vi "Write Result.vi"(0 "Vector Path in":refnum<class "Vector Abstract Path.lvclass">, 11 "error in (no error)":errorcluster) -> (4 "Vector Path out":refnum<class "Vector Abstract Path.lvclass">, 15 "error out":errorcluster)   [LabVIEW 2023, in "RFFixtureCharact.Public.lvlib" / "Vector Abstract Path.lvclass"]
uses:
  Vector Abstract Path.lvclass
  Common/Result Accessor/Result Accessor.lvclass
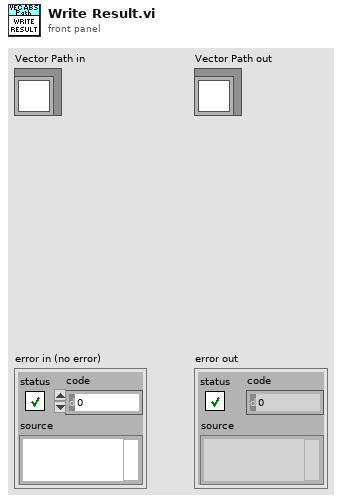
[diagram p1: front panel]
types:
  T1 = typedef "RFFixtureCharact.Public.lvlib/Vector Abstract Path.lvclass/Vector Charact Result.ctl" = cluster{"Port Power":dbl, "Frequency":dbl, "S Parameters":cdb[], "Out Of Limit":bool}
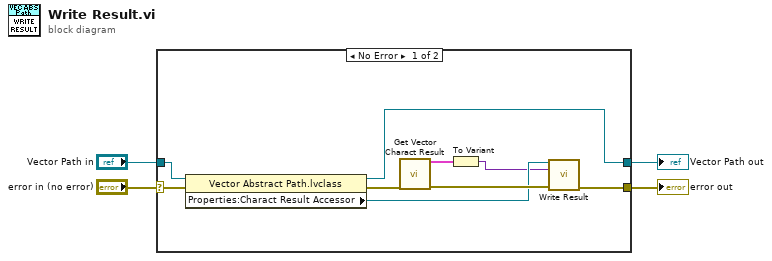
[diagram p0: block diagram]
diagram:
  n1 = case shown="No Error" "error in (no error)" {
    selector: "error in (no error)" -> [w13 w15]
    tunnel: "Vector Path in" -> [w12 w14]
    tunnel: [w8 w15] -> w3
    tunnel: [w10 w14] -> w1
    frame No Error {
      n2 = property class="Vector Abstract Path.lvclass"(reference=w12, error in=w13) -> (reference out=w10:refnum<class "Vector Abstract Path.lvclass">, error out=w11:errorcluster, "Properties:Charact Result Accessor"=w7:refnum<class "Result Accessor.lvclass">)
      n3 = call "Get Vector Charact Result.vi"("error in (no error)"=w11) -> ("Charact Result"=w6:T1[], "error out"=w9:errorcluster)  [unwired: 13 in]
      n4 = To Variant(anything=w6) -> (Variant=w5:variant)
      n5 = call-dynamic "Write Result.vi"("Charact Result Accessor in"=w7, "Charact Result"=w5, "error in"=w9) -> ("error out"=w8:errorcluster)  [unwired: 11 in, 1 out]
    }
    frame Error {
    }
  }
  "error out" <- w3
  "Vector Path out" <- w1
